vi "Data Viewer.vi"(8 "error in":errorcluster, 10 "stop pointer":refnum<class "Pointer.lvclass">, 11 "Server IP Address":string="localhost") -> (0 "error out":errorcluster)   [LabVIEW 2021, in "DSF Core.lvlib"]
uses:
  DSF Core.lvlib
  <vilib>/NI/Memory Manager/Classes/Pointer/Pointer.lvclass
  Source/Main VI/Application Data.ctl
  Source/Buffer Reader/Buffer Data.ctl
  <vilib>/NI/Memory Manager/Classes/Pointer/Read Bool.vi
  <vilib>/NI/Memory Manager/Classes/Pointer/Write Bool.vi
  Typedefs/DSF Settings Info.ctl
  Typedefs/DSF Data Type.ctl
  Typedefs/DSF Byte Order.ctl
  Typedefs/DSF Buffer Type.ctl
  Classes/Thread/Data Server/DSF Buffer Subset Descriptor.ctl
  Source/Buffer Reader/Queue Data.ctl
  Source/Main VI/Values Channels.ctl
  Typedefs/Core Channel Configuration.ctl
  Classes/Configuration/Core/Channel/Channel Configuration.lvclass
  Classes/Configuration/Core/Framework/Framework Configuration.lvclass
  Classes/Configuration/Core/Transfer/Channel Configuration.ctl
  Classes/Configuration/Core/Transfer/Transfer Configuration.lvclass
panel:
  in  "Connect":bool
  out "Connected":bool
  in  "Byte Order":enum16{"big-endian", "little-endian"}(ring)=enum."little-endian"
  in  "Item Tree":string(tree)
  out "Duration":u64 format="%d µs"
  out "Late Count":u64
  out "Iteration":u64
  out "Frequency":dbl format="%.1fHz"
  out "Size":u64 format="%dB"
  out "Decimation":u64
  out "Throughput":dbl format="%_3pB/s"
  out "Values":string
  out "Hex":string
  out "ASCII":string
  # "Data Viewer"
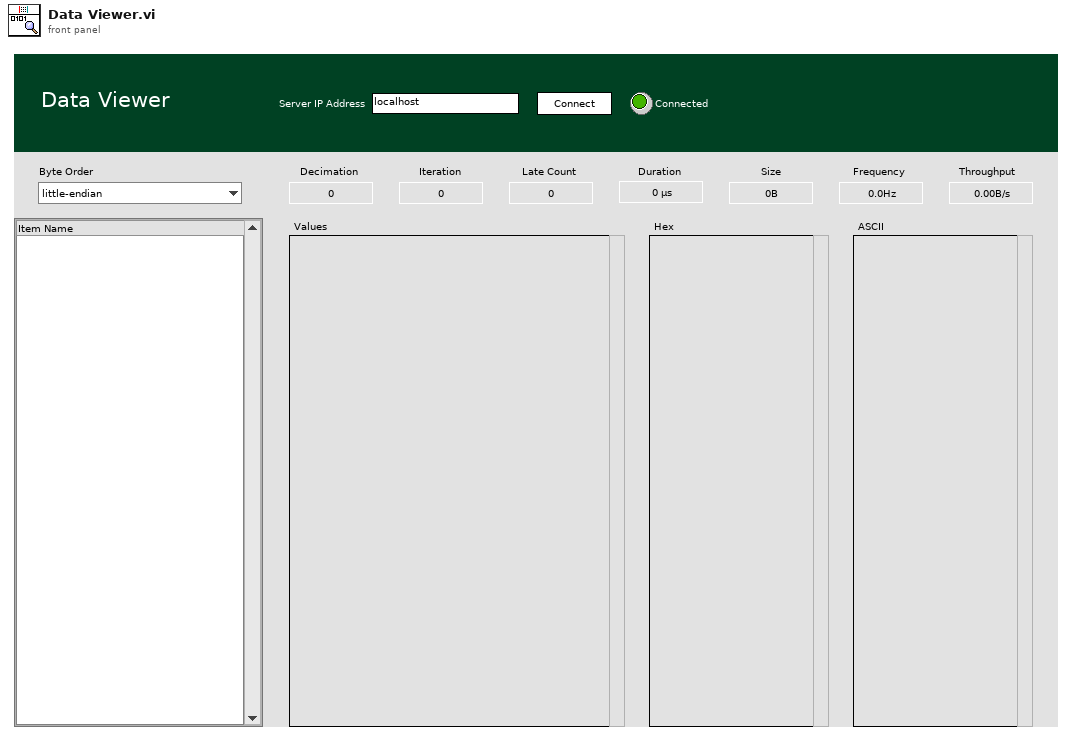
[diagram p1: front panel]
types:
  T1 = typedef "DSF Core.lvlib/Queue Data.ctl" = cluster{"server ID":refnum<k5>, "Buffer data":T2}
  T2 = typedef "DSF Core.lvlib/Buffer Data.ctl" = cluster{"decimation":u64, "avg bandwidth":dbl, "channels":T3[], "byte order":T7, "buffer descriptor":T8, "values channels":T10, "select start offset":u64, "select end offset":u64, "channel index":i32}
  T3 = typedef "DSF Core.lvlib/Transfer Configuration.lvclass/Channel Configuration.ctl" = cluster{"configuration":T4, "component settings":T6[]}
  T4 = typedef "DSF Core.lvlib/Channel Configuration.lvclass/Core Channel Configuration.ctl" = cluster{"name":string, "units":string, "engine data type":T5, "string data type":T5, "string offset":u64}
  T5 = typedef "DSF Core.lvlib/DSF Data Type.ctl" = enum8{"Bool", "SGL", "DBL", "I8", "I16", "I32", "I64", "U8", "U16", "U32", "U64"}
  T6 = typedef "DSF Core.lvlib/DSF Settings Info.ctl" = cluster{"component":string, "values":cluster{"key":string, "value":string}[]}
  T7 = typedef "DSF Core.lvlib/DSF Byte Order.ctl" = enum8{"big-endian", "little-endian"}
  T8 = typedef "DSF Core.lvlib/DSF Buffer Subset Descriptor.ctl" = cluster{"buffer type":T9, "plugin id":i32, "group id":i32, "transfer id":i32, "offset":u64, "length":i64}
  T9 = typedef "DSF Core.lvlib/DSF Buffer Type.ctl" = enum16{"Engine", "String"}
  T10 = typedef "DSF Core.lvlib/Values Channels.ctl" = cluster{"index":i32, "count":i32, "engine offset":u64}
  T11 = typedef "DSF Core.lvlib/Application Data.ctl" = cluster{"Item Tree Control":refnum<vi>, "Top-Level VI":refnum<vi>, "menu reference":refnum<k9>, "queue":refnum<queue>, "Stop Pointer":refnum<class "Pointer.lvclass">, "Buffer Variant":variant, "server ID":refnum<k5>, "framework tag":string, "Values":refnum<vi>, "Hex":refnum<vi>, "ASCII":refnum<vi>, "lines visible":i32, "values padding":i32, "current buffer data":T2, "Framework Configuration":refnum<class "Framework Configuration.lvclass">}
  T12 = typedef "LVPoint32TypeDef.ctl" = cluster{"Horizontal":i32, "Vertical":i32}
  T13 = typedef "DSF Core.lvlib/Data Server Thread.lvclass/Metrics.ctl" = cluster{"framework period":u32, "iteration":u64, "late count":u64, "duration":u64}
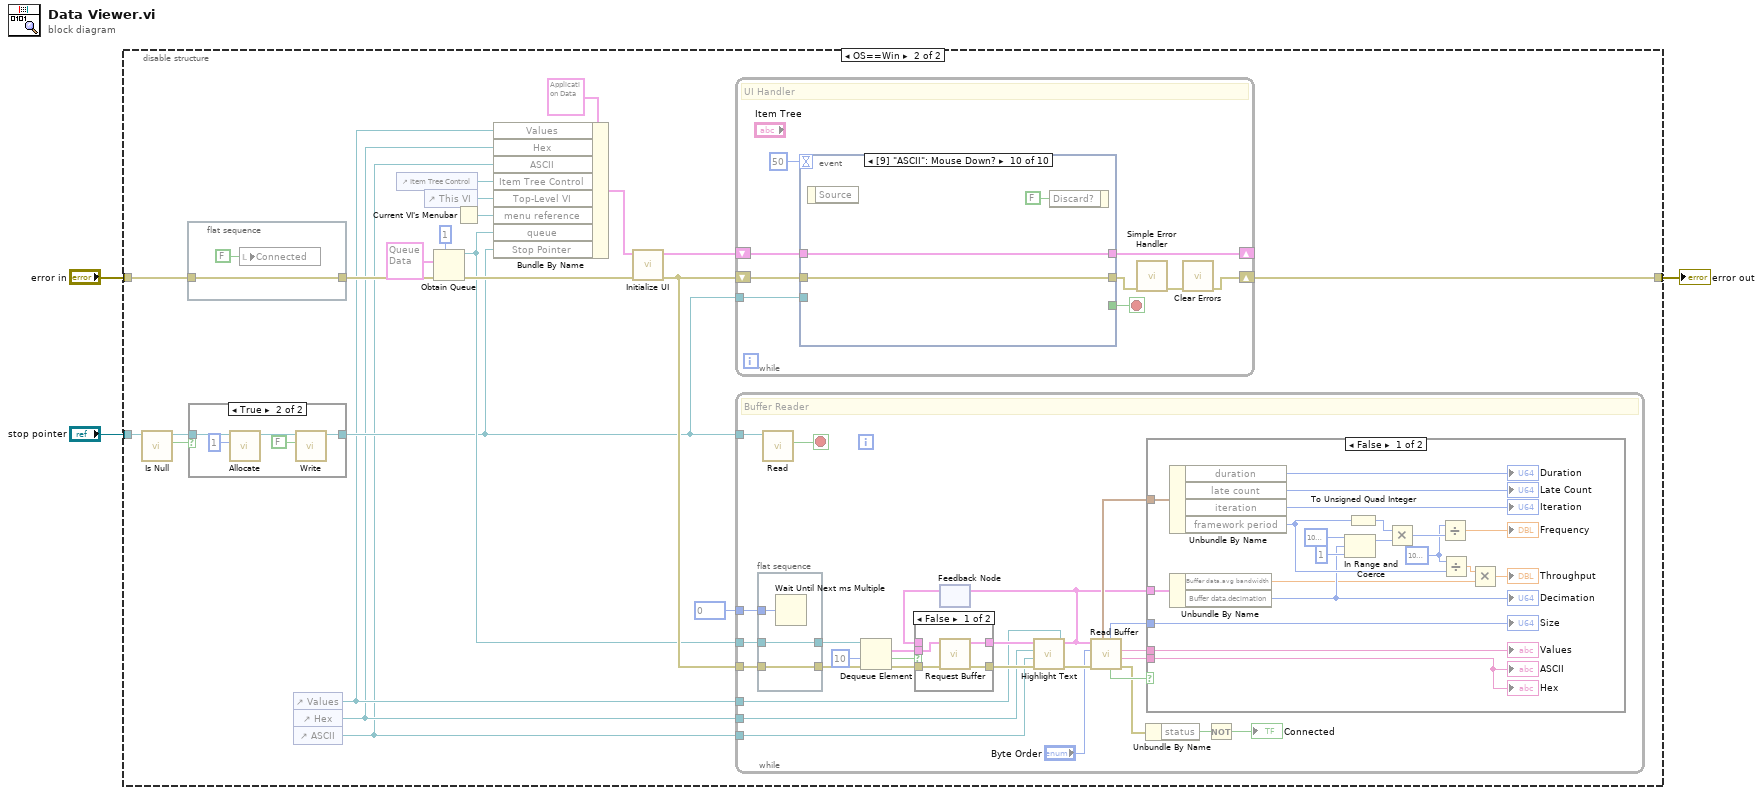
[diagram p0: block diagram]
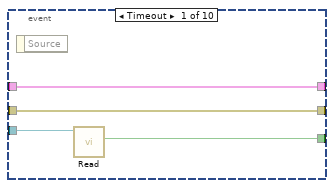
[diagram p6: hidden frame]
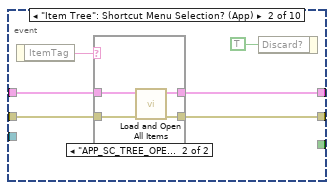
[diagram p7: hidden frame]
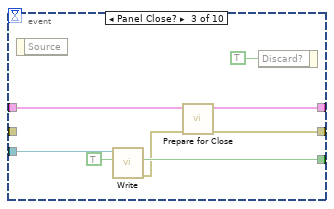
[diagram p9: hidden frame]
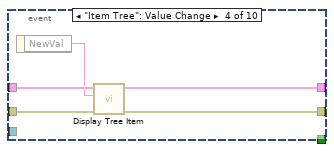
[diagram p10: hidden frame]
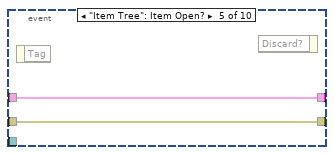
[diagram p11: hidden frame]
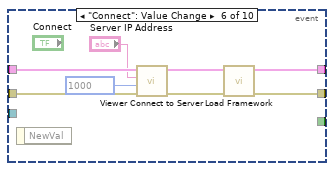
[diagram p12: hidden frame]
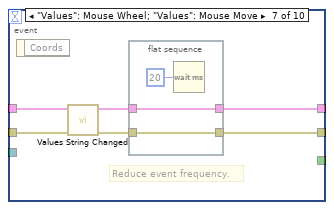
[diagram p13: hidden frame]
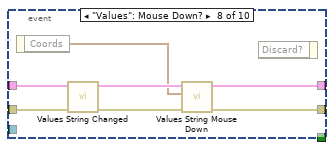
[diagram p14: hidden frame]
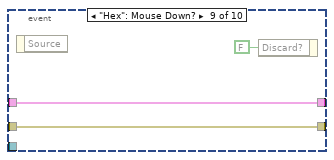
[diagram p15: hidden frame]
diagram:
  n1 = disable-structure shown="OS==Win" {
    disable-tunnel: "error in" -> [w4 w25]
    disable-tunnel: "stop pointer" -> [_ w24]
    disable-tunnel: [w4 w23] -> w1
    frame condition #0 (active) {
    }
    frame condition #1 {
      n2 = call <vilib>:"Is Null.vi"("Pointer in"=w24) -> ("null?"=w15:bool)  [unwired: 8 in, 2 out]
      n3 = flat-sequence {
        tunnel: [w26] -> w10
        tunnel: w25 -> [w26]
        frame #0 {
          n4 = local write "Connected"(FALSE ("Connected")) -> ()
        }
      }
      n5 = case shown="True" w15 {
        tunnel: [w28 w30] -> w9
        tunnel: w24 -> [w28 w32]
        frame False {
        }
        frame True {
          n6 = call <vilib>:"Allocate.vi"("size"=u64 1, "Pointer type"=w32) -> ("Pointer out"=w31:refnum<class "Pointer.lvclass">)  [unwired: 8 in, 1 out]
          n7 = call-poly <vilib>:"Write.vi"("value"=FALSE ("buffer in"), "Pointer in"=w31) -> ("Pointer out"=w30:refnum<class "Pointer.lvclass">)  [unwired: 6 in, 3 out]
        }
      }
      n8 = control-ref of="Values"() -> (w7:refnum<vi>)
      n9 = control-ref of="Hex"() -> (w6:refnum<vi>)
      n10 = control-ref of="ASCII"() -> (w5:refnum<vi>)
      n11 = control-ref of="Item Tree Control"() -> (w19:refnum<vi>)
      n12 = control-ref of="This VI"() -> (w21:refnum<vi>)
      n13 = Obtain Queue(max queue size (-1, unlimited)=1, element data type=T1 {"server ID"=refnum, "Buffer data"={"decimation"=0, "avg bandwidth"=0.0, "channels"=[], "byte order"=enum."little-endian", "buffer descriptor"={"buffer type"=enum."Engine", "plugin id"=0, "group id"=0, "transfer id"=0, "offset"=0, "length"=0}, "values channels"={"index"=0, "count"=0, "engine offset"=0}, "select start offset"=18446744073709551615, "select end offset"=0, "channel index"=-1}} ("Queue data"), error in (no error)=w10) -> (queue out=w11:refnum<queue>, error out=w18:errorcluster)  [unwired: 2 in, 1 out]
      n14 = Current VI's Menubar() -> (w20:refnum<k9>)
      n15 = Bundle By Name(cluster=T11 {"Item Tree Control"=refnum, "Top-Level VI"=refnum, "menu reference"=refnum, "queue"=refnum, "Stop Pointer"=refnum, "Buffer Variant"=variant, "server ID"=refnum, "framework tag"="", "Values"=refnum, "Hex"=refnum, "ASCII"=refnum, "lines visible"=0, "values padding"=0, "current buffer data"={"decimation"=0, "avg bandwidth"=0.0, "channels"=[], "byte order"=enum."big-endian", "buffer descriptor"={"buffer type"=enum."Engine", "plugin id"=0, "group id"=0, "transfer id"=0, "offset"=0, "length"=0}, "values channels"={"index"=0, "count"=0, "engine offset"=0}, "select start offset"=0, "select end offset"=0, "channel index"=0}, "Framework Configuration"=refnum}, "Values"=w7, "Hex"=w6, "ASCII"=w5, "Item Tree Control"=w19, "Top-Level VI"=w21, "menu reference"=w20, "queue"=w11, "Stop Pointer"=w9) -> (w14:T11)
      n16 = call "Initialize UI.vi"("error in (no error)"=w18, "Application Data in"=w14) -> ("error out"=w13:errorcluster, "Application Data out"=w17:T11)  [unwired: 8 in]
      n17 = while {
        shift-right: [w91] -> w23
        shift-left: w13 -> [w99]
        shift-right: [w96] -> _
        shift-left: w17 -> [w95]
        tunnel: w9 -> [w93]
        stop <- w94 stop-if-true
        # "UI Handler"
        n18 = event shown="[9] \"ASCII\": Mouse Down?" {
          selector: _ -> [_ _ _ _ _ _ _ _ _ _]
          dyn-events: _ -> [_ _ _ _ _ _ _ _ _ _]
          timeout: 50 -> [_ _ _ _ _ _ _ _ _ _]
          tunnel: [w100 _ w118 _ _ _ _ _ _ _] -> w94
          tunnel: w99 -> [w103 w106 _ w128 w130 w137 w144 w153 w157 w160]
          tunnel: [w103 w107 w122 w127 w130 w132 w141 w149 w157 w160] -> w97
          tunnel: w95 -> [w102 w108 w116 w125 w129 w138 w143 w154 w156 w159]
          tunnel: [w102 w104 w121 w126 w129 w131 w139 w150 w156 w159] -> w96
          tunnel: w93 -> [w101 _ w120 _ _ _ _ _ _ _]
          event Timeout {
            n19 = event-data() -> ()  [unwired: 1 in, 1 out]
            n20 = call-poly <vilib>:"Read.vi"("Pointer in"=w101) -> ("value out"=w100:bool)  [unwired: 7 in, 3 out]
          }
          event "Item Tree": Shortcut Menu Selection? (App) {
            n21 = event-data() -> ("ItemTag"=w109:string)  [unwired: 1 in]
            n22 = case shown="\"APP_SC_TREE_OPEN_ALL_ITEMS\"" w109 {
              tunnel: w108 -> [w110 w115]
              tunnel: [w111 w113] -> w107
              tunnel: w106 -> [w111 w114]
              tunnel: [w110 w112] -> w104
              frame Default {
              }
              frame "APP_SC_TREE_OPEN_ALL_ITEMS" {
                n23 = call "Load and Open All Items.vi"("error in (no error)"=w114, "Application Data in"=w115) -> ("error out"=w113:errorcluster, "Application Data out"=w112:T11)  [unwired: 8 in]
              }
            }
            n24 = event-data("Discard?"=TRUE) -> ()  [unwired: 1 in, 1 out]
          }
          event Panel Close? {
            n25 = event-data() -> ()  [unwired: 1 in, 1 out]
            n26 = call-poly <vilib>:"Write.vi"("value"=TRUE, "Pointer in"=w120) -> ("error out"=w117:errorcluster, "value"=w118:bool)  [unwired: 6 in, 2 out]
            n27 = call "Prepare for Close.vi"("error in (no error)"=w117, "Application Data in"=w116) -> ("error out"=w122:errorcluster, "Application Data out"=w121:T11)  [unwired: 8 in]
            n28 = event-data("Discard?"=TRUE) -> ()  [unwired: 1 in, 1 out]
          }
          event "Item Tree": Value Change {
            n29 = event-data() -> ("NewVal"=w124:string)  [unwired: 1 in]
            n30 = call "Display Tree Item.vi"("error in (no error)"=w128, "Tag"=w124, "Application Data in"=w125) -> ("error out"=w127:errorcluster, "Application Data out"=w126:T11)  [unwired: 7 in]
          }
          event "Item Tree": Item Open? {
            n31 = event-data() -> ()  [unwired: 1 in, 1 out]
            n32 = event-data() -> ()  [unwired: 2 in, 1 out]
          }
          event "Connect": Value Change {
            n33 = event-data() -> ()  [unwired: 1 in, 1 out]
            n34 = call "Viewer Connect to Server.vi"("error in (no error)"=w137, "timeout ms (60000)"=1000, "server address"="Server IP Address", "Application Refs"=w138) -> ("error out"=w133:errorcluster, "Application Data out"=w134:T11)  [unwired: 6 in]
            n35 = call "Load Framework.vi"("error in (no error)"=w133, "Application Refs"=w134) -> ("error out"=w132:errorcluster, "Application Data out"=w131:T11)  [unwired: 8 in]
          }
          event "Values": Mouse Wheel; "Values": Mouse Move {
            # "Reduce event frequency."
            n36 = event-data() -> ()  [unwired: 1 in, 1 out]
            n37 = call "Values String Changed.vi"("error in (no error)"=w144, "Application Data in"=w143) -> ("error out"=w142:errorcluster, "Application Data out"=w140:T11)  [unwired: 8 in]
            n38 = flat-sequence {
              tunnel: w142 -> [w146]
              tunnel: [w146] -> w141
              tunnel: w140 -> [w145]
              tunnel: [w145] -> w139
              frame #0 {
                n39 = Wait (ms)(milliseconds to wait=u32 20) -> ()  [unwired: 1 out]
              }
            }
          }
          event "Values": Mouse Down? {
            n40 = event-data() -> ("Coords"=w148:T12)  [unwired: 1 in]
            n41 = call "Values String Changed.vi"("error in (no error)"=w153, "Application Data in"=w154) -> ("error out"=w151:errorcluster, "Application Data out"=w152:T11)  [unwired: 8 in]
            n42 = call "Values String Mouse Down.vi"("error in (no error)"=w151, "Coords"=w148, "Application Data in"=w152) -> ("error out"=w149:errorcluster, "Application Data out"=w150:T11)  [unwired: 7 in]
            n43 = event-data() -> ()  [unwired: 2 in, 1 out]
          }
          event "Hex": Mouse Down? {
            n44 = event-data() -> ()  [unwired: 1 in, 1 out]
            n45 = event-data("Discard?"=FALSE) -> ()  [unwired: 1 in, 1 out]
          }
          event "ASCII": Mouse Down? {
            n46 = event-data() -> ()  [unwired: 1 in, 1 out]
            n47 = event-data("Discard?"=FALSE) -> ()  [unwired: 1 in, 1 out]
          }
        }
        n48 = call <vilib>:"Simple Error Handler.vi"("error in (no error)"=w97) -> ("error out"=w98:errorcluster)  [unwired: 4 in, 4 out]
        n49 = call <vilib>:"Clear Errors.vi"("error in (no error)"=w98) -> ("error out"=w91:errorcluster)  [unwired: 5 in, 1 out]
      }
      n50 = while {
        tunnel: w11 -> [w48]
        tunnel: w9 -> [w59]
        tunnel: w13 -> [w47]
        tunnel: u32 0 ("milliseconds to wait") -> [w44]
        tunnel: w5 -> [w36]
        tunnel: w6 -> [w38]
        tunnel: w7 -> [w34]
        stop <- w60 stop-if-true
        # "Buffer Reader"
        n51 = flat-sequence {
          tunnel: w48 -> [w63]
          tunnel: w47 -> [w64]
          tunnel: [w64] -> w45
          tunnel: [w63] -> w46
          tunnel: w44 -> [w62]
          frame #0 {
            n52 = Wait Until Next ms Multiple(millisecond multiple=w62) -> ()  [unwired: 1 out]
          }
        }
        n53 = call-poly <vilib>:"Read.vi"("Pointer in"=w59) -> ("value out"=w60:bool)  [unwired: 7 in, 3 out]
        n54 = Dequeue Element(queue=w46, timeout in ms (-1)=10, error in (no error)=w45) -> (element=w55:T1, timed out?=w54:bool, error out=w56:errorcluster)  [unwired: 1 out]
        n55 = feedback #1() -> (w53:T1)  [unwired: 1 in]
        n56 = case shown="False" w54 {
          tunnel: w56 -> [w68 w69]
          tunnel: w55 -> [w67 _]
          tunnel: [w66 w69] -> w42
          tunnel: [w65 w70] -> w41
          tunnel: w53 -> [_ w70]
          frame False {
            n57 = call "Request Buffer.vi"("error in (no error)"=w68, "queue data in"=w67) -> ("error out"=w66:errorcluster, "queue data out"=w65:T1)  [unwired: 8 in]
          }
          frame True {
          }
        }
        n58 = call "Highlight Text.vi"("Values"=w34, "error in (no error)"=w42, "ASCII"=w36, "Hex"=w38, "queue data in"=w41) -> ("error out"=w40:errorcluster, "queue data out"=w39:T1)  [unwired: 5 in]
        n59 = feedback-in #1(w39) -> ()
        n60 = call "Read Buffer.vi"("error in"=w40, "byte order (little-endian)"="Byte Order", "queue data in"=w39) -> ("error out"=w37:errorcluster, "buffer data"=w57:string, "values string"=w43:string, "timed out?"=w51:bool, "buffer size"=w58:u64, "metrics"=w49:T13)  [unwired: 2 in, 1 out]
        n61 = Unbundle By Name(w37) -> ("status"=w52:bool)
        n62 = case shown="False" w51 {
          tunnel: w58 -> [w85 _]
          tunnel: w43 -> [w84 _]
          tunnel: w57 -> [w83 _]
          tunnel: w49 -> [w80 _]
          tunnel: w39 -> [w79 _]
          frame False {
            w72 = u64 1000000 ("y")
            n63 = Unbundle By Name(w80) -> ("duration"=→"Duration":u64, "late count"=→"Late Count":u64, "iteration"=→"Iteration":u64, "framework period"=w75:u32)
            n64 = Unbundle By Name(w79) -> ("Buffer data.avg bandwidth"=w71:dbl, "Buffer data.decimation"=w74:u64)
            "Decimation" <- w74
            n65 = In Range and Coerce(upper limit=u64 1000000 ("lower limit"), x=w74, lower limit=u64 1) -> (coerced(x)=w86:u64)  [unwired: 1 out]
            n66 = To Unsigned Quad Integer(1:w75) -> (0:w88:u64)
            n67 = Multiply(x=w88, y=w86) -> (x*y=w90:u64)
            n68 = Divide(x=w72, y=w90) -> (x/y=→"Frequency":dbl)
            n69 = Divide(x=w72, y=w75) -> (x/y=w73:dbl)
            n70 = Multiply(x=w73, y=w71) -> (x*y=→"Throughput":dbl)
            "Hex" <- w83
            "Size" <- w85
            "ASCII" <- w83
            "Values" <- w84
          }
          frame True {
          }
        }
        n71 = Not(x=w52) -> (.not. x?=→"Connected":bool)
      }
    }
  }
  "error out" <- w1
